vi "Engine Simulation Globals.vi"() -> ()   [LabVIEW 2010]
panel:
  out "Engine Speed":fxp<+/-,47,-4> format="%.54g"
  in  "EngineSim Global Reset":bool
  in  "ECU Event Cycles to Filter":u16
  in  "Cam Half Speed?":bool
  out "Cycle Angle":fxp<+,61,10>
  out "Crank Tooth Width":fxp<+,61,10>
  out "Crank Angle":fxp<+,60,9> format="%.54g"
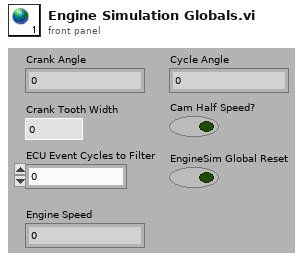
[diagram p1: front panel]
diagram:
